vi "GUI Interlock Tester-setup.vi"(8 "Self Test Button":refnum<vi>, 9 "Power Off Button":refnum<vi>, 10 "Power On Button":refnum<vi>, 11 "test case ID":string) -> (0 "Self Test Button out":refnum<vi>, 1 "Power Off Button out":refnum<vi>, 2 "Power On Button out":refnum<vi>, 3 "Power State":bool)   [LabVIEW 2018]
doc: "The setup VI should be executed before the VI under test in the harness VI. In this VI you can prepare the environment and the inputs of the VI under test.\n\nSee the Help Document for more information. (<b>Help</b> > <b>IncQuery Labs</b> > <b>InstaCoverage</b> > <b>InstaCoverage Help...</b>)"
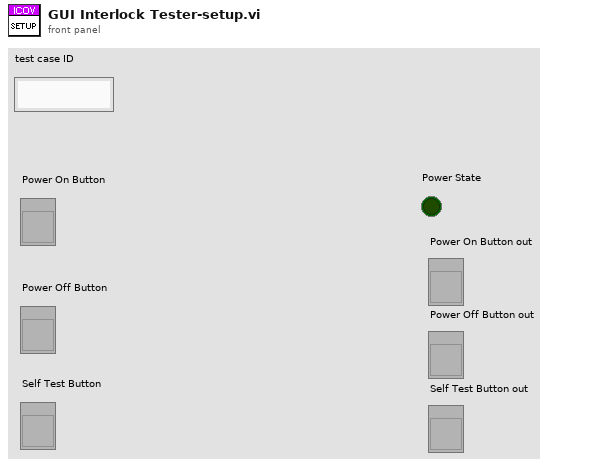
[diagram p1: front panel]
types:
  T1 = enum8{"Enabled", "Disabled", "Disabled and Grayed Out"}
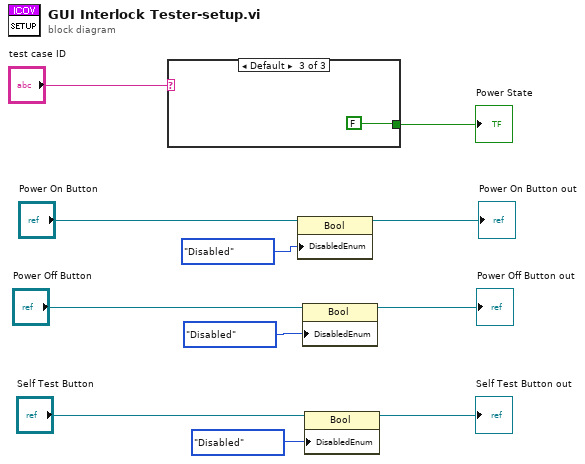
[diagram p0: block diagram]
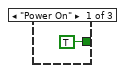
[diagram p2: hidden frame]
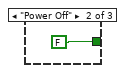
[diagram p3: hidden frame]
diagram:
  n1 = case shown="Default" "test case ID" {
    tunnel: [TRUE FALSE FALSE] -> w10
    frame "Power On" {
    }
    frame "Power Off" {
    }
    frame Default {
    }
  }
  "Power State" <- w10
  n2 = property class="Bool"(reference="Power On Button", "DisabledEnum"=T1."Disabled" ("Disabled")) -> (reference out=→"Power On Button out":refnum<vi>)  [unwired: 1 in, 1 out]
  n3 = property class="Bool"(reference="Power Off Button", "DisabledEnum"=T1."Disabled" ("Disabled")) -> (reference out=→"Power Off Button out":refnum<vi>)  [unwired: 1 in, 1 out]
  n4 = property class="Bool"(reference="Self Test Button", "DisabledEnum"=T1."Disabled" ("Disabled")) -> (reference out=→"Self Test Button out":refnum<vi>)  [unwired: 1 in, 1 out]
